vi "braces.vi"(10 "Numeric":i32) -> (2 "spaces":string)   [LabVIEW 2019, in "Userlib.lvlib"]
uses:
  Userlib.lvlib
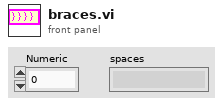
[diagram p1: front panel]
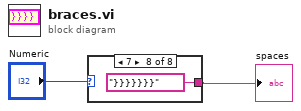
[diagram p0: block diagram]
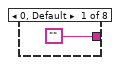
[diagram p2: hidden frame]
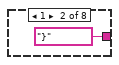
[diagram p3: hidden frame]
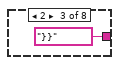
[diagram p4: hidden frame]
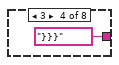
[diagram p5: hidden frame]
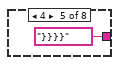
[diagram p6: hidden frame]
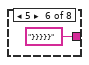
[diagram p7: hidden frame]
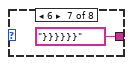
[diagram p8: hidden frame]
diagram:
  n1 = case shown="7" "Numeric" {
    tunnel: ["" "}" ("space") "}}" ("space") "}}}" ("space") "}}}}" ("space") "}}}}}" ("space") "}}}}}}" ("space") "}}}}}}}" ("space")] -> w2
    frame 0, Default {
    }
    frame 1 {
    }
    frame 2 {
    }
    frame 3 {
    }
    frame 4 {
    }
    frame 5 {
    }
    frame 6 {
    }
    frame 7 {
    }
  }
  "spaces" <- w2
